vi "AutoDuringTeleop.vi"(11 "error in":errorcluster) -> ()   [LabVIEW 2020]
uses:
  AutoDuringTeleopRoutines.ctl
  <vilib>/Rock Robotics/WPI/Framework/Command Status Info.ctl
  <vilib>/Rock Robotics/WPI/Framework/Completion Status.ctl
  <vilib>/Rock Robotics/WPI/Framework/Completion Notifier.ctl
  Framework/Robot Global Data.vi
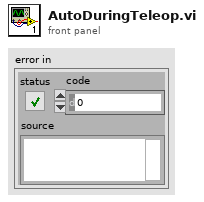
[diagram p1: front panel]
types:
  T1 = typedef "AutoDuringTeleopRoutines.ctl" = enum16{"None", "1", "2", "3"}
  T2 = typedef "Command Status Info.ctl" = cluster{"Name":string, "Status":T3, "notifier out":T4}
  T3 = typedef "Completion Status.ctl" = enum16{"Successful", "Aborted", "Incomplete"}
  T4 = typedef "Completion Notifier.ctl" = refnum<notifier>
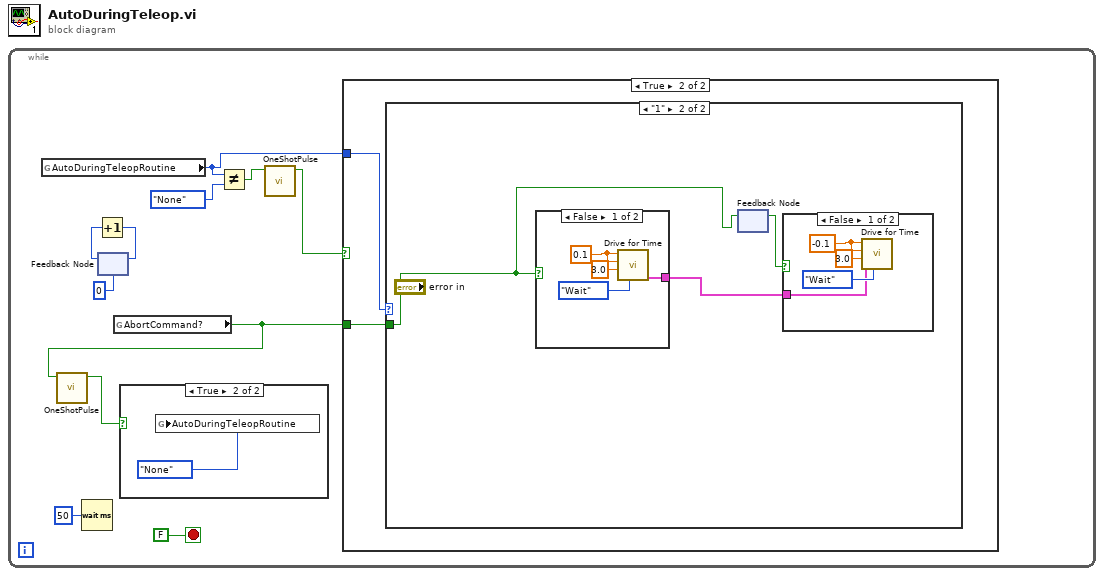
[diagram p0: block diagram]
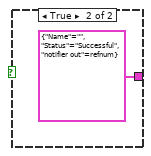
[diagram p6: hidden frame]
diagram:
  n1 = while {
    stop <- FALSE stop-if-true
    n2 = global read "Robot Global Data.vi" "AutoDuringTeleopRoutine"() -> (w6:enum16{"None", "1", "2", "3"})
    n3 = Wait (ms)(milliseconds to wait=u32 50) -> ()  [unwired: 1 out]
    n4 = feedback #1(0) -> (w2:i32)
    n5 = Increment(x=w2) -> (x+1=w1:i32)
    n6 = feedback-in #1(w1) -> ()
    n7 = global read "Robot Global Data.vi" "AbortCommand?"() -> (w5:bool)
    n8 = call "OneShotPulse.vi"("Input"=w5) -> ("Output"=w4:bool)  [unwired: 10 in]
    n9 = case shown="True" w4 {
      frame False {
      }
      frame True {
        n10 = global write "Robot Global Data.vi" "AutoDuringTeleopRoutine"(AutoDuringTeleopRoutines."None" ("Enum")) -> ()
      }
    }
    n11 = Not Equal?(x=w6, y=AutoDuringTeleopRoutines."None" ("Enum")) -> (x != y?=w8:bool)
    n12 = call "OneShotPulse.vi"("Input"=w8) -> ("Output"=w7:bool)  [unwired: 10 in]
    n13 = case shown="True" w7 {
      tunnel: w6 -> [_ w14]
      tunnel: w5 -> [_ w13]
      frame False {
      }
      frame True {
        n14 = case shown="\"1\"" w14 {
          tunnel: w13 -> [_ w16]
          frame "None", Default {
          }
          frame "1" {
            n15 = case shown="False" w16 {
              tunnel: [w22 T2 {"Name"="", "Status"=enum."Successful", "notifier out"=refnum} ("Command Info Out")] -> w17
              frame False {
                w25 = 0.1 ("Left Speed")
                n16 = call "Drive for Time.vi"("Synchronization"=enum16{"Start", "Wait"}."Wait", "Seconds"=3.0, "Right Speed"=w25, "Left Speed"=w25) -> ("Command Info Out"=w22:T2)  [unwired: 7 in]
              }
              frame True {
              }
            }
            n17 = feedback-in #2(w16) -> ()
            n18 = feedback #2() -> (w15:bool)  [unwired: 1 in]
            n19 = case shown="False" w15 {
              tunnel: w17 -> [w18 _]
              frame False {
                w21 = -0.1 ("Left Speed")
                n20 = call "Drive for Time.vi"("Synchronization"=enum16{"Start", "Wait"}."Wait", "Command Info In"=w18, "Seconds"=3.0, "Right Speed"=w21, "Left Speed"=w21) -> ()  [unwired: 6 in, 1 out]
              }
              frame True {
              }
            }
          }
        }
      }
    }
  }
